vi "Single Clothoid Calculation.vi"(9 "Angle":dbl, 10 "Min R":dbl) -> (3 "Zeroes out":T1)   [LabVIEW 2018]
uses:
  BlendType.ctl
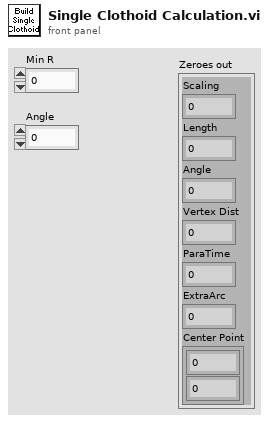
[diagram p1: front panel]
types:
  T1 = typedef "BlendType.ctl" = cluster{"Scaling":dbl, "Length":dbl, "Angle":dbl, "Vertex Dist":dbl, "ParaTime":dbl, "ExtraArc":dbl, "Center Point":cluster{dbl, dbl}}
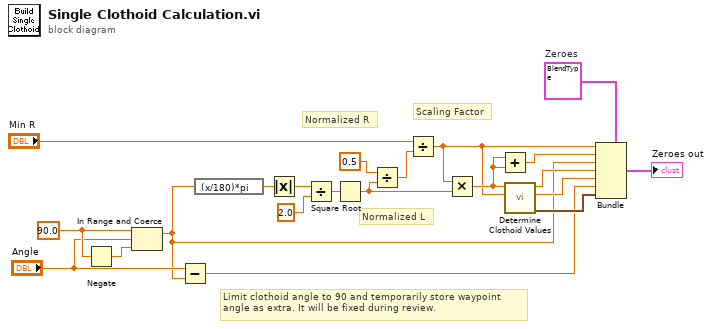
[diagram p0: block diagram]
diagram:
  w5 = 90.0
  w6 = T1 {"Scaling"=0.0, "Length"=0.0, "Angle"=0.0, "Vertex Dist"=0.0, "ParaTime"=0.0, "ExtraArc"=0.0, "Center Point"={0.0, 0.0}}  # Zeroes
  # "Limit clothoid angle to 90 and temporarily store waypoint\nangle as extra. It will be fixed during review."
  # "Normalized L"
  # "Scaling Factor"
  # "Normalized R"
  n1 = Negate(x=w5) -> (-x=w19:dbl)
  n2 = In Range and Coerce(upper limit=w5, x="Angle", lower limit=w19) -> (coerced(x)=w3:dbl)  [unwired: 1 out]
  n3 = Subtract(x="Angle", y=w3) -> (x-y=w1:dbl)
  n4 = expression code="(x/180)*pi" ("radians to degrees")(w3) -> (w2:dbl)
  n5 = Absolute Value(x=w2) -> (abs(x)=w14:dbl)
  n6 = Divide(x=w14, y=2.0) -> (x/y=w10:dbl)
  n7 = Square Root(x=w10) -> (sqrt(x)=w20:dbl)
  n8 = Divide(x=0.5, y=w20) -> (x/y=w8:dbl)
  n9 = Divide(x="Min R", y=w8) -> (x/y=w16:dbl)
  n10 = Multiply(x=w16, y=w20) -> (x*y=w17:dbl)
  n11 = Add(x=w17, y=w17) -> (x+y=w18:dbl)
  n12 = call "Determine Clothoid Values.vi"("Scaling"=w16, "Desired Length"=w17) -> ("Center Point"=w21:cluster{dbl, dbl}, "Para Time"=w13:dbl, "Vertex Dist ft"=w15:dbl)  [unwired: 6 in, 1 out]
  n13 = Bundle(cluster=w6, "Scaling"=w16, "Length"=w18, "Angle"=w3, "Vertex Dist"=w15, "ParaTime"=w13, "ExtraArc"=w1, "Center Point"=w21) -> (→"Zeroes out":T1)
